vi "Sub_serial_delay_and_Read_byte.vi"(8 "에러 입력(에러 없음)":errorcluster, 10 "Delay(1000ms)":u32=1000, 11 "VISA 참조 번호 입력":refnum<visa-resource-name>) -> (0 "에러 출력":errorcluster, 2 "버퍼 읽기":string, 3 "VISA 참조 번호 출력":refnum<visa-resource-name>)   [LabVIEW 2015]
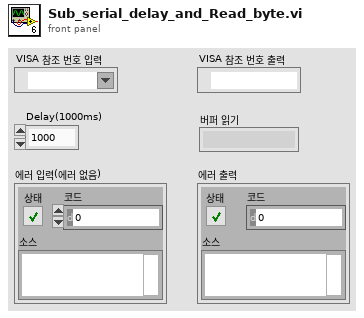
[diagram p1: front panel]
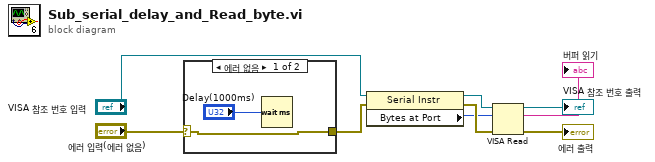
[diagram p0: block diagram]
diagram:
  n1 = case shown="에러 없음" "에러 입력(에러 없음)" {
    selector: "에러 입력(에러 없음)" -> [w10 w12]
    tunnel: [w10 w12] -> w8
    frame No Error {
      n2 = Wait (ms)(milliseconds to wait="Delay(1000ms)") -> ()  [unwired: 1 out]
    }
    frame Error {
    }
  }
  n3 = property class="Serial Instr"(reference="VISA 참조 번호 입력", error in=w8) -> (reference out=w3:refnum<visa-resource-name>, error out=w6:errorcluster, "Bytes at Port"=w2:u32)
  n4 = VISA Read(VISA resource name=w3, byte count=w2, error in (no error)=w6) -> (VISA resource name out=→"VISA 참조 번호 출력":refnum<visa-resource-name>, read buffer=→"버퍼 읽기":string, error out=→"에러 출력":errorcluster)  [unwired: 1 out]
